vi "Initialize.vi"(8 "error in (no error)":errorcluster, 11 "MFC in":refnum<class "Valve.lvclass">) -> (0 "error out":errorcluster, 3 "MFC out":refnum<class "Valve.lvclass">)   [LabVIEW 2013, in "Valve.lvlib" / "Valve.lvclass"]
uses:
  Valve.lvclass
  Valve.lvclass/Valve.ctl
  Read Valve Position.vi
  Write VISA.vi
  <vilib>/Instr/_visa.llb/VISA Configure Serial Port (Instr).vi
  PluginInterface/PluginInterface.lvlibp/PluginInterfaceClass/Read TDMS File Path.vi
  PluginInterface/PluginInterface.lvlibp/PluginInterfaceClass/Read DVR.vi
  PluginInterface/PluginInterface.lvlibp/PluginInterfaceClass/Write TDMS.vi
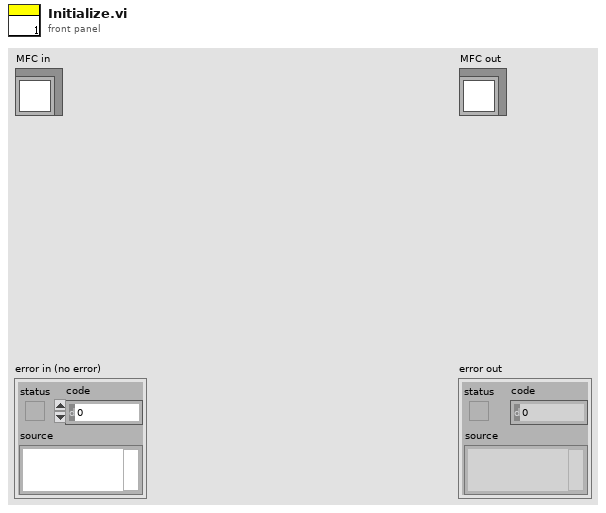
[diagram p1: front panel]
types:
  T1 = enum16{"open", "open or create", "create or replace", "create", "open (read-only)"}
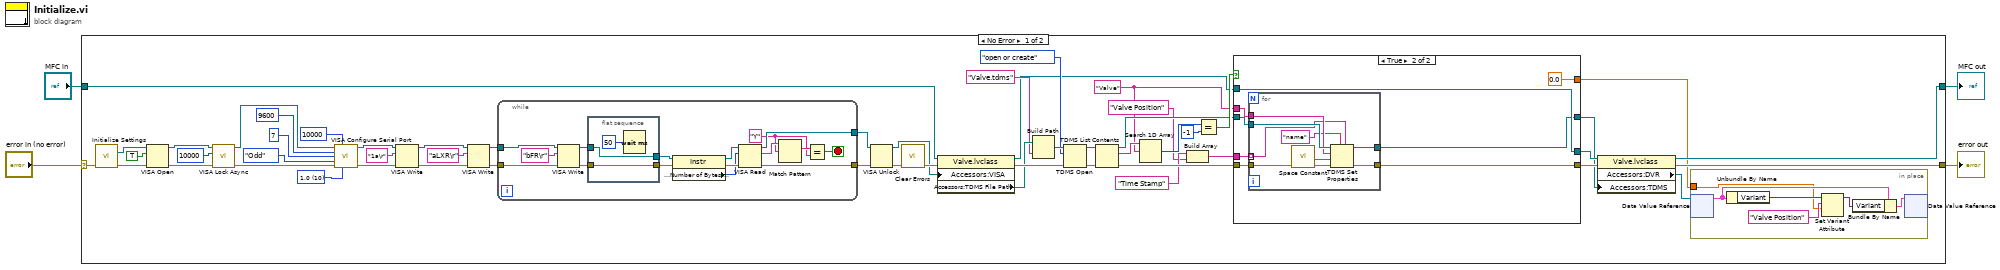
[diagram p0: block diagram]
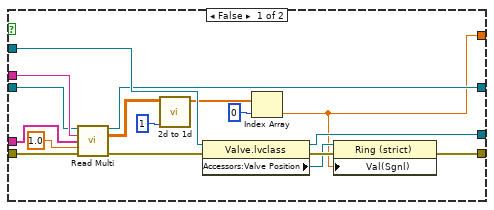
[diagram p2: hidden frame]
diagram:
  n1 = case shown="No Error" "error in (no error)" {
    selector: "error in (no error)" -> [w38 w117]
    tunnel: [w33 w117] -> w3
    tunnel: [w34 w116] -> w1
    tunnel: "MFC in" -> [w9 w116]
    frame No Error {
      w23 = u16 10 items=["1.0"=10, "1.5"=15, "2.0"=20] ("stop bits (10: 1 bit)")
      w51 = "Valve"
      n2 = call "Initialize Settings.vi"("error in (no error)"=w38) -> ("VISA resource name 2"=w13:refnum<visa-resource-name>, "error out"=w12:errorcluster)  [unwired: 13 in]
      n3 = VISA Open(duplicate session (F)=TRUE, error in (no error)=w12, VISA resource name=w13) -> (VISA resource name=w28:refnum<visa-resource-name>, error out=w29:errorcluster)  [unwired: 2 in]
      n4 = call <vilib>:"VISA Lock Async.vi"("error in (no error)"=w29, "timeout (0)"=u32 10000, "VISA resource name"=w28) -> ("error out"=w14:errorcluster, "VISA resource name out"=w15:refnum<visa-resource-name>)  [unwired: 6 in, 1 out]
      n5 = call-poly "VISA Configure Serial Port"("VISA resource name"=w15, "timeout (10sec)"=u32 10000, "baud rate (9600)"=u32 9600, "data bits (8)"=u16 7, "parity (0:none)"=enum16{"None", "Odd", "Even", "Mark", "Space"}."Odd", "error in (no error)"=w14, "stop bits (10: 1 bit)"=w23) -> ("VISA resource name out"=w16:refnum<visa-resource-name>, "error out"=w17:errorcluster)  [unwired: 2 in, 5 out]
      n6 = VISA Write(VISA resource name=w16, write buffer="1a\r", error in (no error)=w17) -> (VISA resource name out=w19:refnum<visa-resource-name>, error out=w18:errorcluster)  [unwired: 1 out]
      n7 = VISA Write(VISA resource name=w19, write buffer="aLXR\r", error in (no error)=w18) -> (VISA resource name out=w7:refnum<visa-resource-name>, error out=w8:errorcluster)  [unwired: 1 out]
      n8 = while {
        tunnel: w8 -> [w63]
        tunnel: [w70] -> w32
        tunnel: [w69] -> w31
        tunnel: w7 -> [w58]
        stop <- w65 stop-if-true
        w66 = "Y" ("regular expression")
        n9 = VISA Write(VISA resource name=w58, write buffer="bFR\r", error in (no error)=w63) -> (VISA resource name out=w62:refnum<visa-resource-name>, error out=w60:errorcluster)  [unwired: 1 out]
        n10 = flat-sequence {
          tunnel: [w75] -> w61
          tunnel: w62 -> [w75]
          tunnel: [w74] -> w59
          tunnel: w60 -> [w74]
          frame #0 {
            n11 = Wait (ms)(milliseconds to wait=u32 50) -> ()  [unwired: 1 out]
          }
        }
        n12 = property class="Instr"(reference=w61, error in=w59) -> (reference out=w73:refnum<visa-resource-name>, error out=w72:errorcluster, "Serial Settings:Number of Bytes at Serial Port"=w71:u32)
        n13 = VISA Read(VISA resource name=w73, byte count=w71, error in (no error)=w72) -> (VISA resource name out=w70:refnum<visa-resource-name>, read buffer=w68:string, error out=w69:errorcluster)  [unwired: 1 out]
        n14 = Match Pattern(string=w68, regular expression=w66) -> (match substring=w67:string)  [unwired: 1 in, 3 out]
        n15 = Equal?(x=w67, y=w66) -> (x = y?=w65:bool)
      }
      n16 = VISA Unlock(8:w31, 11:w32) -> (0:w11:errorcluster, 3:w10:refnum<visa-resource-name>)
      n17 = call <vilib>:"Clear Errors.vi"("error in (no error)"=w11) -> ("error out"=w47:errorcluster)  [unwired: 6 in]
      n18 = property class="Valve.lvclass"(reference=w9, error in=w47, "Accessors:VISA"=w10) -> (reference out=w39:refnum<class "Valve.lvclass">, error out=w45:errorcluster, "Accessors:TDMS File Path"=w42:path)
      n19 = Build Path(base path=w42, name or relative path="Valve.tdms") -> (appended path=w46:path)
      n20 = TDMS Open(8:w45, 10:T1."open or create" ("operation (0:open)"), 11:w46) -> (0:w44:errorcluster, 3:w40:refnum<k34>)  [unwired: 4 in]
      n21 = TDMS List Contents(4:w44, 7:w40) -> (0:w52:errorcluster, 2:w55:string[], 3:w53:refnum<k34>)  [unwired: 1 in, 1 out]
      n22 = Search 1D Array(1D array=w55, element=w51) -> (index of element=w56:i32)  [unwired: 1 in]
      n23 = Build Array("Time Stamp" ("Channel"), "Valve Position" ("string")) -> (w50:string[])
      n24 = Equal?(x=w56, y=-1) -> (x = y?=w54:bool)
      n25 = case shown="True" w54 {
        tunnel: w53 -> [w94 w107]
        tunnel: [w85 w103] -> w36
        tunnel: w52 -> [w97 w105]
        tunnel: w51 -> [w98 w106]
        tunnel: w39 -> [w99 w102]
        tunnel: w50 -> [w86 w104]
        tunnel: [w93 w102] -> w35
        tunnel: [w84 w101] -> w6
        tunnel: [w83 0.0 ("Numeric Control")] -> w5
        frame False {
          n26 = call "Read Multi.vi"("tdms file in"=w94, "group"=w98, "Channel"=w86, "Numeric"=1.0, "error in (no error)"=w97) -> ("tdms file out"=w84:refnum<k34>, "Array"=w91:dbl[][], "error out"=w96:errorcluster)  [unwired: 7 in, 1 out]
          n27 = call "2d to 1d.vi"("index"=1, "array"=w91) -> ("output array"=w90:dbl[])  [unwired: 9 in]
          n28 = property class="Valve.lvclass"(reference=w99, error in=w96) -> (reference out=w93:refnum<class "Valve.lvclass">, error out=w89:errorcluster, "Accessors:Valve Position"=w88:refnum<vi>)
          n29 = Index Array(array=w90, index=0) -> (element=w83:dbl)
          n30 = property class="Ring (strict)"(reference=w88, error in=w89, "Val(Sgnl)"=w83) -> (error out=w85:errorcluster)  [unwired: 1 out]
        }
        frame True {
          n31 = for {
            tunnel: w105 -> [w115]
            tunnel: [w114] -> w103
            tunnel: w107 -> [w113]
            tunnel: w106 -> [w112]
            tunnel: w104 -> [w111] mode=indexing
            tunnel: [w108] -> w101
            n32 = call <vilib>:"Space Constant.vi"() -> ("String"=w109:string)
            n33 = TDMS Set Properties(5:w111, 7:"name" ("property names"), 8:w115, 9:w109, 10:w112, 11:w113) -> (0:w114:errorcluster, 3:w108:refnum<k34>)  [unwired: 2 out]
          }
        }
      }
      n34 = property class="Valve.lvclass"(reference=w35, error in=w36, "Accessors:TDMS"=w6) -> (reference out=w34:refnum<class "Valve.lvclass">, error out=w33:errorcluster, "Accessors:DVR"=w37:refnum<data-value>)
      n35 = in-place {
        in-place-border: w5 -> [w77]
        n36 = in-place-dvr #1(w37) -> (w79:cluster{"Array":string[], "Variant":variant})  [unwired: 1 out]
        n37 = Unbundle By Name(w79) -> ("Variant"=w81:variant)
        n38 = Set Variant Attribute(Variant=w81, name="Valve Position" ("string"), value=w77) -> (Variant out=w80:variant)  [unwired: 1 in, 2 out]
        n39 = Bundle By Name(cluster=w79, "Variant"=w80) -> (w82:cluster{"Array":string[], "Variant":variant})
        n40 = in-place-dvr #1(w82) -> ()  [unwired: 2 out]
      }
    }
    frame Error {
    }
  }
  "error out" <- w3
  "MFC out" <- w1
